vi "CALC_omega(w)_(arr).vi"(8 "Twisted neck (F)":bool, 9 "Alt. magnets orientation (F)":bool, 10 "abs(theta) < pi, rad":dbl[](array[numeric]), 11 "theta, rad":dbl[](array[numeric])) -> (3 "w, deg":dbl[](array[numeric]))   [LabVIEW 2018, in "Tracker.lvlib"]
uses:
  Tracker.lvlib
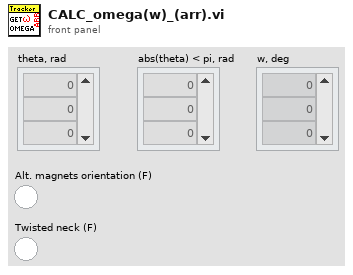
[diagram p1: front panel]
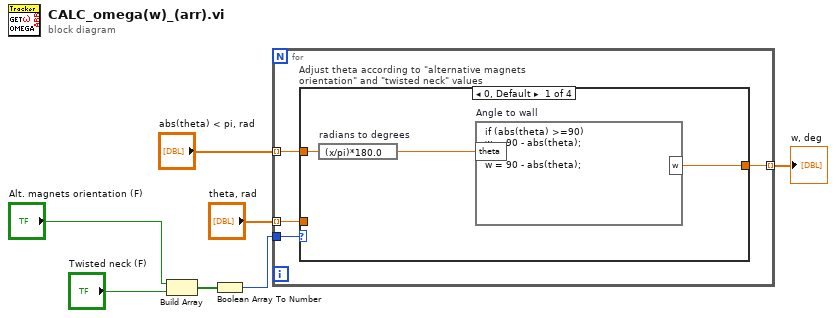
[diagram p0: block diagram]
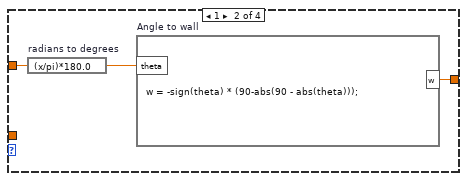
[diagram p2: hidden frame]
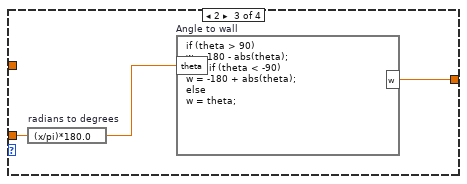
[diagram p3: hidden frame]
diagram:
  n1 = Build Array("Alt. magnets orientation (F)", "Twisted neck (F)") -> (w4:bool[])
  n2 = Boolean Array To Number(Boolean array=w4) -> (number=w3:u32)
  n3 = for {
    tunnel: "theta, rad" -> [w11] mode=indexing
    tunnel: [w10] -> w6 mode=indexing
    tunnel: "abs(theta) < pi, rad" -> [w9] mode=indexing
    tunnel: w3 -> [w8]
    n4 = case "Adjust theta according to \"alternative magnets orientation\" and \"twisted neck\" values" shown="0, Default" w8 {
      tunnel: w9 -> [w13 w16 _ w21]
      tunnel: [w14 w17 w20 w21] -> w10
      tunnel: w11 -> [_ _ w19 _]
      frame 0, Default {
        n5 = expression code="(x/pi)*180.0" "radians to degrees"(w13) -> (w12:dbl)
        n6 = formula code="if (abs(theta) >=90)\nw = 90 - abs(theta);\nelse\nw = 90 - abs(theta);" "Angle to wall"("theta"=w12) -> ("w"=w14:dbl)
      }
      frame 1 {
        n7 = expression code="(x/pi)*180.0" "radians to degrees"(w16) -> (w15:dbl)
        n8 = formula code="w = -sign(theta) * (90-abs(90 - abs(theta)));" "Angle to wall"("theta"=w15) -> ("w"=w17:dbl)
      }
      frame 2 {
        n9 = expression code="(x/pi)*180.0" "radians to degrees"(w19) -> (w18:dbl)
        n10 = formula code="if (theta > 90)\nw = 180 - abs(theta);\nelse if (theta < -90)\nw = -180 + abs(theta);\nelse\nw = theta;" "Angle to wall"("theta"=w18) -> ("w"=w20:dbl)
      }
      frame 3 {
      }
    }
  }
  "w, deg" <- w6
